vi "initialize.vi"(8 "error in":errorcluster, 9 "Timeout (ms)":i32=-1, 10 "device (if slave)":u8, 11 "profibus reference":T1) -> (0 "error out":errorcluster, 3 "profibus reference out":T1)   [LabVIEW 2013, in "dynamic profibus.lvlib"]
uses:
  dynamic profibus.lvlib
  fpga reference.ctl
  profibus master action.ctl
  <vilib>/rvi/interface/common/niFpgaWaitOnOcc.vi
  <vilib>/Utility/error.llb/Error Cluster From Error Code.vi
  <vilib>/rvi/errors/niLvFpgaAdjustHostInterfaceError.vi
  <vilib>/rvi/interface/nirviMethod/nirviMethod.xnode
  <vilib>/FPGAPlugInAG/Dynamic/niLvFpga_WriteFifo_Dynamic.vi
  <vilib>/rvi/errors/niLvFpgaMergeErrorWithErrorCode.vi
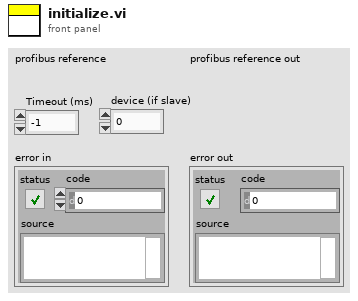
[diagram p1: front panel]
types:
  T1 = typedef "dynamic profibus.lvlib/fpga reference.ctl" = refnum<k20>
  T2 = typedef "dynamic profibus.lvlib/profibus master action.ctl" = enum8{"initialize", "uninitialize", "stop", "get input", "get input size", "set output", "get output size", "get diagnostic", "transfer data", "transfer diagnostics"}
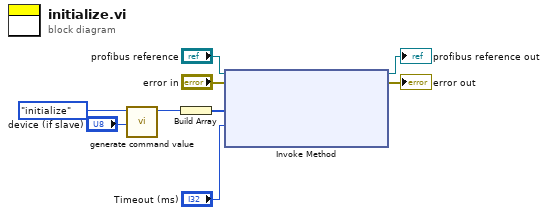
[diagram p0: block diagram]
diagram:
  n1 = call "generate command value.vi"("device"="device (if slave)", "action"=profibus_master_action."initialize") -> ("Element"=w4:u32)  [unwired: 9 in]
  n2 = Build Array(w4) -> (w3:u32[])
  n3 = xnode "Invoke Method"("FPGA VI Reference In"="profibus reference", "error in"="error in", "Data"=w3, "Timeout (ms)"="Timeout (ms)") -> ("FPGA VI Reference Out"=→"profibus reference out":T1, "error out"=→"error out":errorcluster)  [unwired: 1 out]
